vi "rawpathToInterp.vi"(8 "error in (no error)":errorcluster, 10 "create interp img folder":bool=TRUE, 11 "Path":path) -> (0 "error out":errorcluster, 1 "Angle lineout path":path, 2 "Spectrum lineout path":path, 3 "Interpolated image path":path)   [LabVIEW 2020]
panel:
  out "Interp folder":path
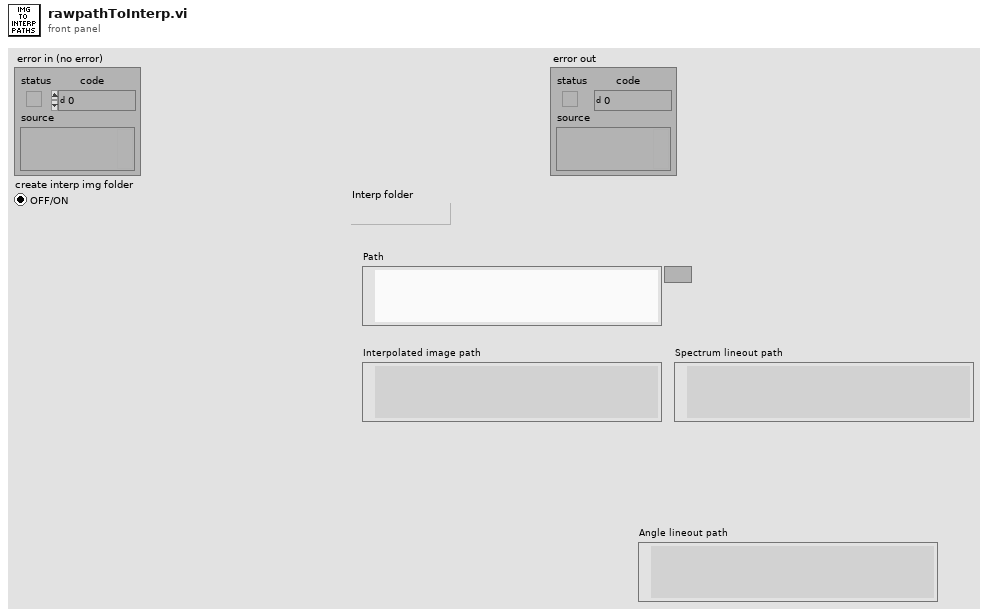
[diagram p1: front panel]
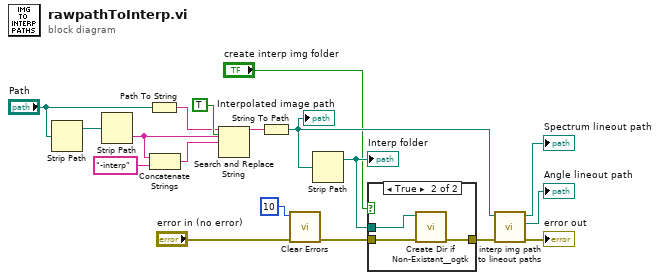
[diagram p0: block diagram]
diagram:
  n1 = Strip Path(path="Path") -> (stripped path=w17:path)  [unwired: 1 out]
  n2 = Strip Path(path=w17) -> (name=w14:string)  [unwired: 1 out]
  n3 = Path To String(path="Path") -> (string=w15:string)
  n4 = Concatenate Strings(w14, "-interp") -> (w10:string)
  n5 = Search and Replace String(replace all?=TRUE ("replace all? (F)"), input string=w15, search string=w14, replace string=w10) -> (result string=w12:string)  [unwired: 4 in, 3 out]
  n6 = String To Path(string=w12) -> (path=w5:path)
  "Interpolated image path" <- w5
  n7 = call <vilib>:"Clear Errors.vi"("error in (no error)"="error in (no error)", "specific error code to clear (0: all)"=10) -> ("error out"=w1:errorcluster)  [unwired: 4 in, 1 out]
  n8 = Strip Path(path=w5) -> (stripped path=w7:path)  [unwired: 1 out]
  "Interp folder" <- w7
  n9 = case shown="True" "create interp img folder" {
    tunnel: w7 -> [_ w22]
    tunnel: w1 -> [w19 w21]
    tunnel: [w19 w20] -> w6
    frame False {
    }
    frame True {
      n10 = call <userlib>:"Create Dir if Non-Existant__ogtk.vi"("error in (no error)"=w21, "Directory Path"=w22) -> ("error out"=w20:errorcluster)  [unwired: 7 in, 2 out]
    }
  }
  n11 = call "interp img path to lineout paths.vi"("error in (no error)"=w6, "Interp image path"=w5) -> ("error out"=→"error out":errorcluster, "angle lineout path"=→"Angle lineout path":path, "Spectrum lineout path"=→"Spectrum lineout path":path)  [unwired: 7 in]
